vi "Encoder_004.vi"(10 "Image Path":path, 11 "Encoder parameters":T1) -> (1 "v(t)":dbl(graph), 2 "Total # spikes":i32, 3 "Input":dbl, 4 "spike indexes":i32[](array[numeric]), 6 "total duration":i32, 7 "Picture":picture)   [LabVIEW 2018]
panel:
  out "1-bit pixmap":bool[][](array[boolean])
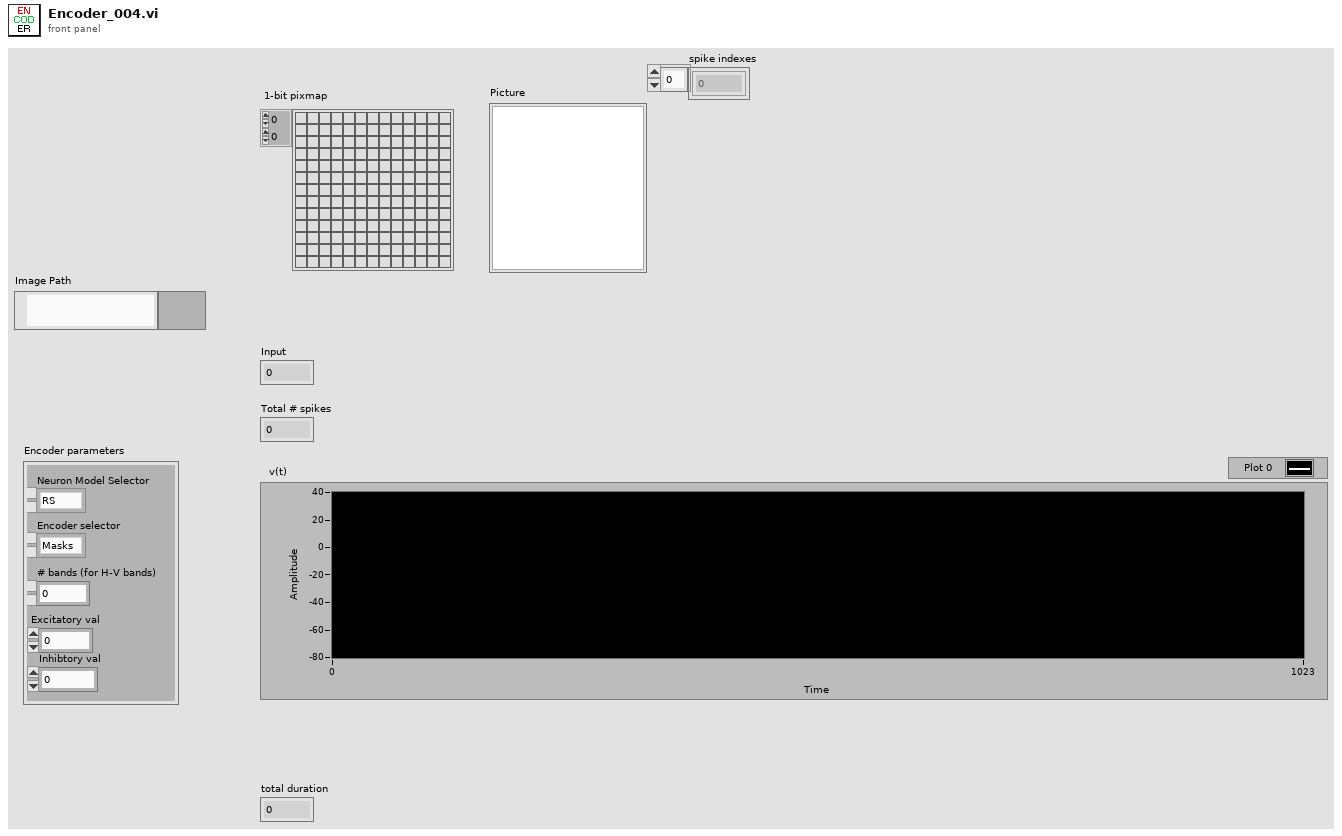
[diagram p1: front panel]
types:
  T1 = cluster{"Encoder selector":enum16{"Masks", "H-V bands", "Simple reading"}, "# bands (for H-V bands)":i32, "Excitatory val":dbl, "Inhibtory val":dbl, "Neuron Model Selector":enum16{"RS", "LTS", "RZ", "TC2", "TC1", "FS", "CH", "IB"}}
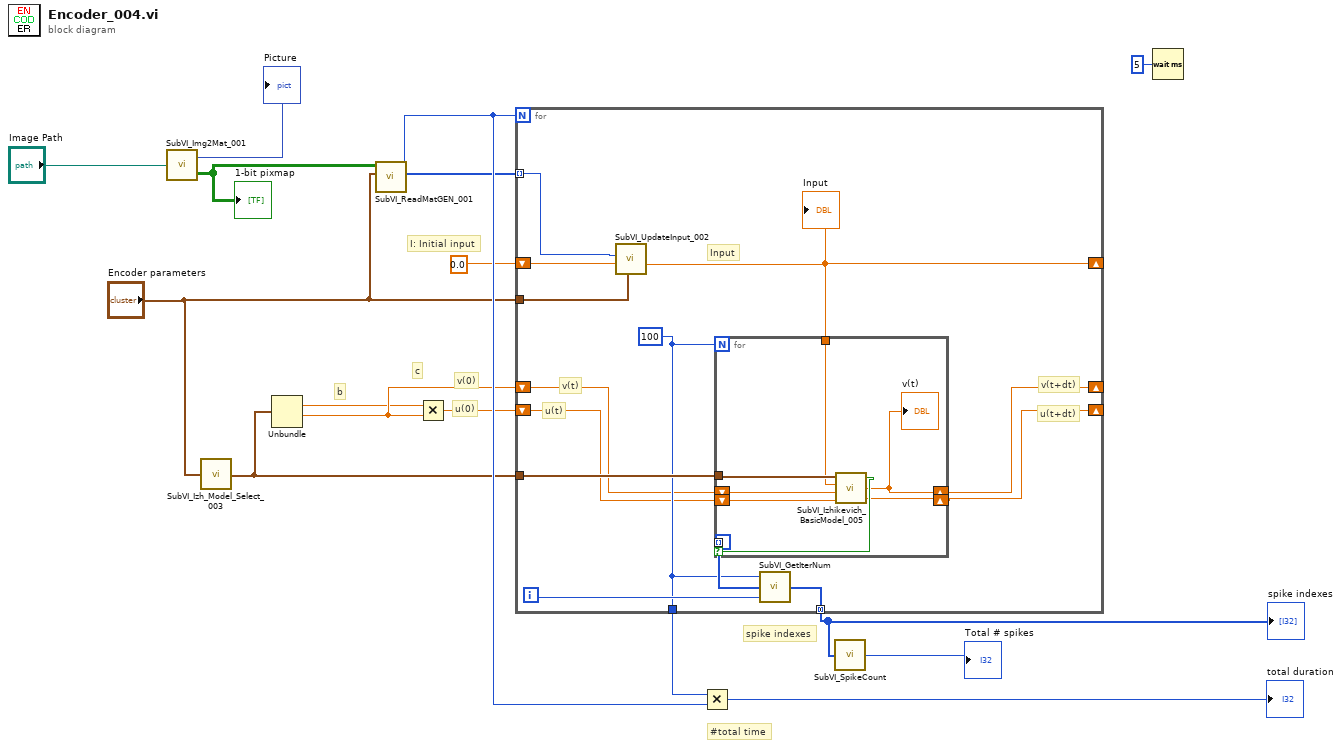
[diagram p0: block diagram]
diagram:
  # "#total time"
  # "spike indexes"
  # "v(0)"
  # "c"
  # "b"
  # "u(0)"
  # "I: Initial input"
  n1 = call "SubVI_Img2Mat_001.vi"("Path"="Image Path") -> ("Picture"=→"Picture":picture, "1-bit pixmap"=w5:bool[][])
  "1-bit pixmap" <- w5
  n2 = call "SubVI_Izh_Model_Select_003.vi"("Encoder parameters"="Encoder parameters") -> ("output cluster"=w12:cluster{dbl, dbl, dbl, dbl})
  n3 = Unbundle(w12) -> (w9:dbl, w10:dbl)  [unwired: 2 out]
  n4 = call "SubVI_ReadMatGEN_001.vi"("Encoder parameters 2"="Encoder parameters", "1-bit pixmap   in"=w5) -> ("array of inputs"=w4:i32[], "total #iter"=w14:i32)  [unwired: 8 in]
  n5 = Multiply(x=w9, y=w10) -> (x*y=w8:dbl)
  n6 = for {
    N: w14 -> [_]
    tunnel: w4 -> [w22] mode=indexing
    shift-right: [w27] -> _
    shift-left: 0.0 ("x") -> [w29]
    shift-right: [w19] -> _
    shift-left: w8 -> [w17]
    shift-right: [w20] -> _
    shift-left: w10 -> [w18]
    tunnel: w12 -> [w28]
    tunnel: [w24] -> w2 mode=concatenating
    tunnel: "Encoder parameters" -> [w21]
    tunnel: [w23] -> w13
    i -> [w25]
    w23 = 100
    # "v(t+dt)"
    # "u(t+dt)"
    # "v(t)"
    # "u(t)"
    # "Input"
    n7 = call "SubVI_UpdateInput_002.vi"("Encoder parameters"=w21, "Previous Input (in)"=w29, "New info"=w22) -> ("Input (out)"=w27:dbl)  [unwired: 8 in]
    "Input" <- w27
    n8 = for {
      N: w23 -> [_]
      tunnel: w28 -> [w36]
      tunnel: w27 -> [w35]
      tunnel: [w37] -> w26 mode=indexing if=w34
      shift-right: [w33] -> w20
      shift-left: w18 -> [w31]
      shift-right: [w32] -> w19
      shift-left: w17 -> [w30]
      i -> [w37]
      n9 = call "SubVI_Izhikevich_BasicModel_005.vi"("u(t)"=w30, "v(0)"=w31, "I"=w35, "Model parameters"=w36) -> ("u(t+dt)"=w32:dbl, "v(t+dt)"=w33:dbl, "Spike?"=w34:bool)
      "v(t)" <- w33
    }
    n10 = call "SubVI_GetIterNum.vi"("#iter outer loop"=w25, "#iter inner loop"=w26, "N inner loop"=w23) -> ("#iter GLOBAL"=w24:i32[])
  }
  "spike indexes" <- w2
  n11 = Multiply(x=w13, y=w14) -> (x*y=→"total duration":i32)
  n12 = call "SubVI_SpikeCount.vi"("Spike index input"=w2) -> ("Total # spikes"=→"Total # spikes":i32)
  n13 = Wait (ms)(milliseconds to wait=u32 5) -> ()  [unwired: 1 out]
